vi "niDTS WLAN UTIL CH BW to Hz.vi"(10 "CH BW":T1) -> (2 "CH BW Hz":dbl format="%#_6p")   [LabVIEW 2015, in "niDTS WLAN.lvlib"]
uses:
  niDTS WLAN.lvlib
  Includes/niDTS WLAN INC CH BW.ctl
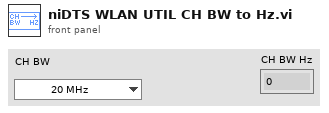
[diagram p1: front panel]
types:
  T1 = typedef "niDTS WLAN.lvlib/niDTS WLAN INC CH BW.ctl" = enum16{"20 MHz", "40 MHz", "80 MHz", "160 MHz"}
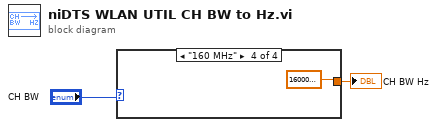
[diagram p0: block diagram]
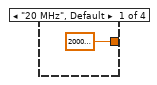
[diagram p2: hidden frame]
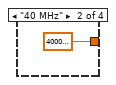
[diagram p3: hidden frame]
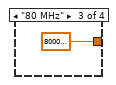
[diagram p4: hidden frame]
diagram:
  n1 = case shown="\"160 MHz\"" "CH BW" {
    tunnel: [20000000.0 40000000.0 80000000.0 160000000.0] -> w1
    frame "20 MHz", Default {
    }
    frame "40 MHz" {
    }
    frame "80 MHz" {
    }
    frame "160 MHz" {
    }
  }
  "CH BW Hz" <- w1
